vi "Set Enable Debugging.vi"(8 "error in (no error)":errorcluster, 9 "Wait for debugger on launch (false)":bool, 10 "Enable debugging (false)":bool, 11 "PPL in":refnum<class "NI_AB_API_DPPL.lvclass">) -> (0 "error out":errorcluster, 3 "PPL out":refnum<class "NI_AB_API_DPPL.lvclass">)   [LabVIEW 2020, in "NI_AB_API_DPPL.lvclass"]
uses:
  <vilib>/AppBuilder/AB_API/DPPL/NI_AB_API_DPPL.lvclass
  <vilib>/AppBuilder/AB_API/PPL/NI_AB_API_PPL.lvclass
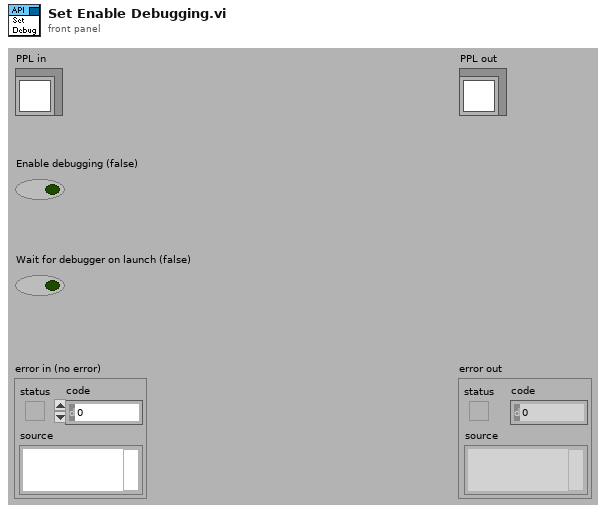
[diagram p1: front panel]
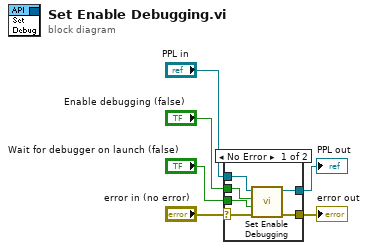
[diagram p0: block diagram]
diagram:
  n1 = case shown="No Error" "error in (no error)" {
    selector: "error in (no error)" -> [w10 w14]
    tunnel: [w9 w14] -> w5
    tunnel: [w11 w13] -> w3
    tunnel: "PPL in" -> [w12 w13]
    tunnel: "Enable debugging (false)" -> [w8 _]
    tunnel: "Wait for debugger on launch (false)" -> [w7 _]
    frame No Error {
      n2 = call-parent "Set Enable Debugging.vi"("error in (no error)"=w10, "Wait for debugger on launch (false)"=w7, "Enable debugging (false)"=w8, "PPL in"=w12) -> ("error out"=w9:errorcluster, "PPL out"=w11:refnum<class "NI_AB_API_DPPL.lvclass">)  [unwired: 6 in]
    }
    frame Error {
    }
  }
  "error out" <- w5
  "PPL out" <- w3
